vi "Unit Discrete Delay (Poly).vi"   [LabVIEW 2011]
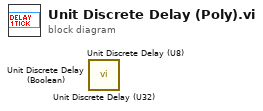
[diagram p0: block diagram]
diagram:
  n1 = call <userlib>:"Unit Discrete Delay (U32).vi"() -> ()  [unwired: 15 in, 1 out]
  n2 = call <userlib>:"Unit Discrete Delay (U8).vi"() -> ()  [unwired: 15 in, 1 out]
  n3 = call <userlib>:"Unit Discrete Delay (Boolean).vi"() -> ()  [unwired: 15 in, 1 out]
